vi "Sequencing.vi"(1 "error in":T1) -> ()   [LabVIEW 2014]
uses:
  ErrorOut.ctl
  Robot Global Data.vi
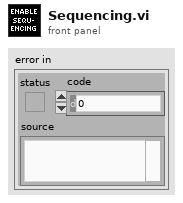
[diagram p1: front panel]
types:
  T1 = typedef "ErrorOut.ctl" = errorcluster
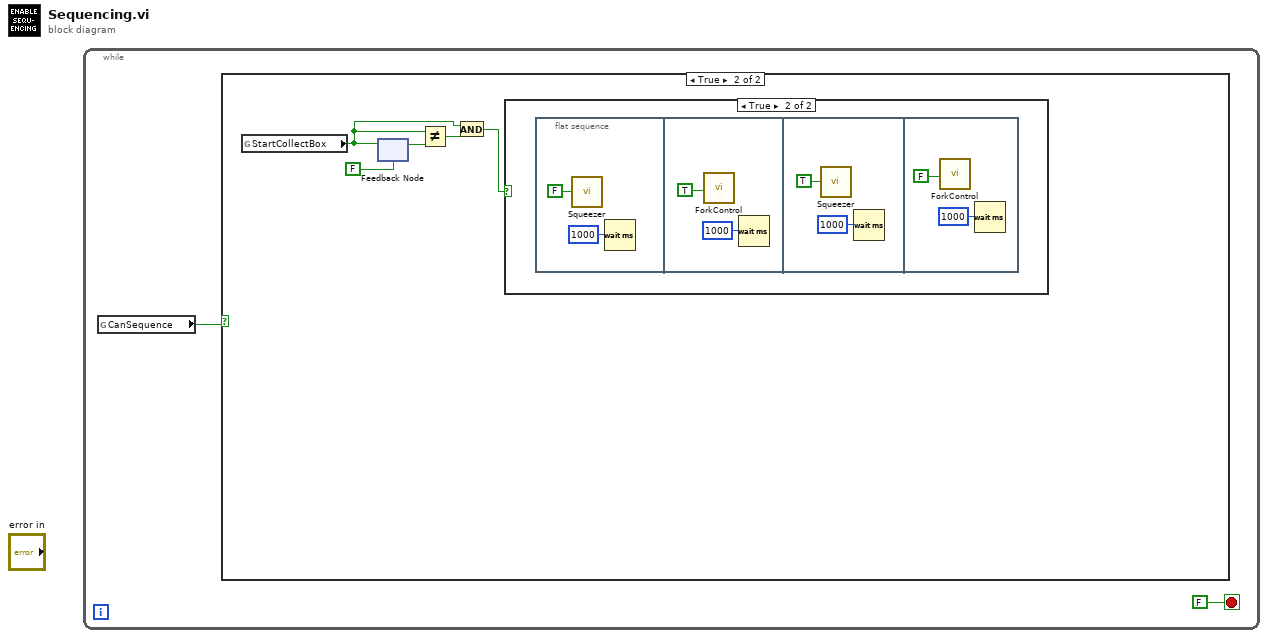
[diagram p0: block diagram]
diagram:
  n1 = while {
    stop <- FALSE stop-if-true
    n2 = global read "Robot Global Data.vi" "CanSequence"() -> (w1:bool)
    n3 = case shown="True" w1 {
      frame False {
      }
      frame True {
        n4 = global read "Robot Global Data.vi" "StartCollectBox"() -> (w4:bool)
        n5 = feedback-in #1(w4) -> ()
        n6 = feedback #1(FALSE) -> (w6:bool)
        n7 = Not Equal?(x=w4, y=w6) -> (x != y?=w5:bool)
        n8 = And(x=w4, y=w5) -> (x .and. y?=w3:bool)
        n9 = case shown="True" w3 {
          frame False {
          }
          frame True {
            n10 = flat-sequence {
              frame #0 {
                n11 = call "Squeezer.vi"("Direction"=FALSE) -> ()
                n12 = Wait (ms)(milliseconds to wait=u32 1000) -> ()  [unwired: 1 out]
              }
              frame #1 {
                n13 = call "ForkControl.vi"("Direction"=TRUE) -> ()
                n14 = Wait (ms)(milliseconds to wait=u32 1000) -> ()  [unwired: 1 out]
              }
              frame #2 {
                n15 = call "Squeezer.vi"("Direction"=TRUE) -> ()
                n16 = Wait (ms)(milliseconds to wait=u32 1000) -> ()  [unwired: 1 out]
              }
              frame #3 {
                n17 = call "ForkControl.vi"("Direction"=FALSE) -> ()
                n18 = Wait (ms)(milliseconds to wait=u32 1000) -> ()  [unwired: 1 out]
              }
            }
          }
        }
      }
    }
  }
